vi "Determine Warnings.vi"(9 "Min Temp":dbl, 10 "Max Temp":dbl, 11 "Current Temp":dbl) -> (1 "Warning?":bool, 2 "Warning Text":string)   [LabVIEW 2010]
doc: "This VI is the solution to an exercise in LabVIEW Core I. It is used to determine the string to output to the weather station based on the current temperature and limit settings.\n\nInputs: Current Temp (DBL), Min Temp (DBL), and Max Temp (DBL).\nOutputs: Warning Text (string) and Warning? (Boolean)."
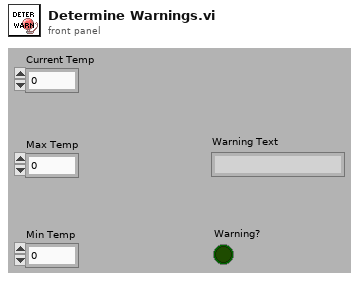
[diagram p1: front panel]
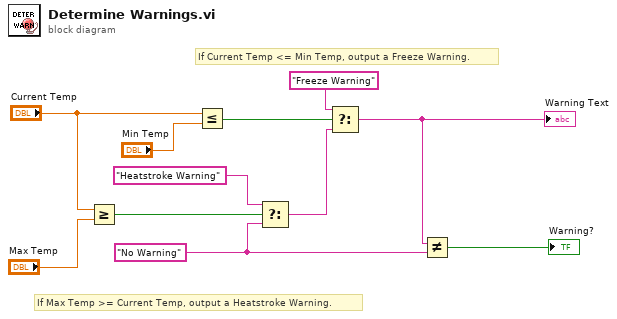
[diagram p0: block diagram]
diagram:
  w1 = "No Warning" ("f")
  # "If Current Temp <= Min Temp, output a Freeze Warning."
  # "If Max Temp >= Current Temp, output a Heatstroke Warning."
  n1 = Greater Or Equal?(x="Current Temp", y="Max Temp") -> (x >= y?=w8:bool)
  n2 = Less Or Equal?(x="Current Temp", y="Min Temp") -> (x <= y?=w3:bool)
  n3 = Select(t="Heatstroke Warning", s=w8, f=w1) -> (s? t:f=w2:string)
  n4 = Select(t="Freeze Warning", s=w3, f=w2) -> (s? t:f=w11:string)
  "Warning Text" <- w11
  n5 = Not Equal?(x=w11, y=w1) -> (x != y?=→"Warning?":bool)
